vi "clear_IRQ_data.vi"(1 "error IO":errorcluster) -> (0 "error IO 2":errorcluster)   [LabVIEW 2021]
uses:
  ISRglobals.vi
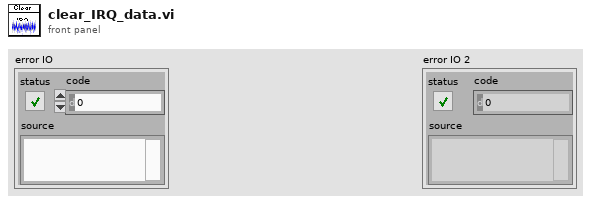
[diagram p1: front panel]
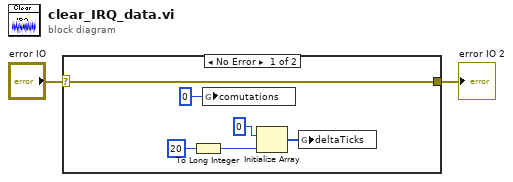
[diagram p0: block diagram]
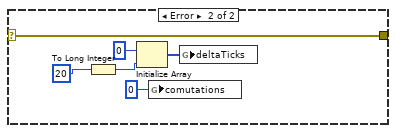
[diagram p2: hidden frame]
diagram:
  n1 = case shown="No Error" "error IO" {
    selector: "error IO" -> [w7 w14]
    tunnel: [w7 w14] -> w1
    frame No Error {
      n2 = To Long Integer(number=20) -> (32bit integer=w4:i32)
      n3 = global write "ISRglobals.vi" "comutations"(i64 0 ("comutations")) -> ()
      n4 = Initialize Array(i64 0, w4) -> (w5:i64[])
      n5 = global write "ISRglobals.vi" "deltaTicks"(w5) -> ()
    }
    frame Error {
      n6 = To Long Integer(number=20) -> (32bit integer=w10:i32)
      n7 = Initialize Array(i64 0, w10) -> (w11:i64[])
      n8 = global write "ISRglobals.vi" "comutations"(i64 0 ("comutations")) -> ()
      n9 = global write "ISRglobals.vi" "deltaTicks"(w11) -> ()
    }
  }
  "error IO 2" <- w1
